vi "Update All Values.vi"(8 "error in (no error)":errorcluster, 10 "Values":refnum<class "Type.lvclass">[](array[class]), 11 "Entity in":refnum<class "Entity.lvclass">) -> (0 "error out":errorcluster, 3 "Entity out":refnum<class "Entity.lvclass">)   [LabVIEW 2022 SP3, in "Conditum.lvlib" / "Entity.lvclass"]
uses:
  Entity.lvclass
  Entity.lvclass/Entity.ctl
  Columns/Type/Type.lvclass
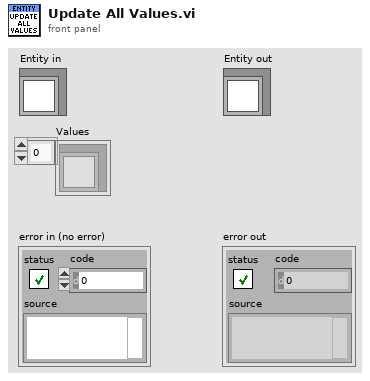
[diagram p1: front panel]
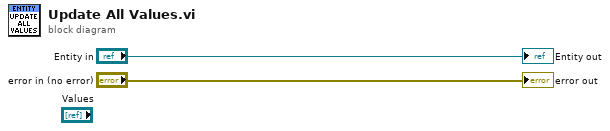
[diagram p0: block diagram]
diagram:
  "error out" <- "error in (no error)"
  "Entity out" <- "Entity in"
